vi "2D Auto Correlation (DBL).vi"(11 "X":dbl[][](array[numeric])) -> (0 "error":i32, 3 "Rxx":dbl[][](array[numeric]))   [LabVIEW 2017, in "NI_AALPro.lvlib"]
doc: "Computes the autocorrelation of the input sequence <B>X</B>. Wire data to the <B>X</B> input to determine the polymorphic instance to use or manually select the instance."
uses:
  <vilib>/Analysis/NI_AALPro.lvlib
  <resource>/lvanlys.dll
panel:
  # "2D AutoCorrelation (DBL)"
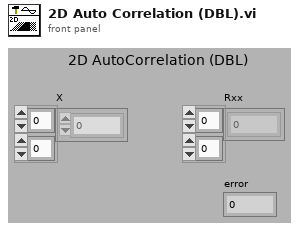
[diagram p1: front panel]
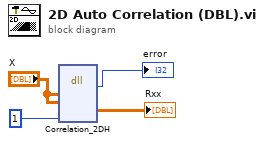
[diagram p0: block diagram]
diagram:
  n1 = dll-call lib="e:/builds/penguin/labview/branches/2017/dev/dist/resource/lvanlys.*" fn="Correlation_2DH"("xH"="X", "yH"="X", "domain"=1 ("conv_corr")) -> (→"error":i32, "rxyH"=→"Rxx":dbl[][])  [unwired: 7 in, 2 out]
